vi "Init from Ref.vi"(8 "error in":errorcluster, 10 "Cell Ref":refnum<k24>, 11 "Image in":refnum<class "Image.lvclass">) -> (0 "error out":errorcluster, 3 "Image out":refnum<class "Image.lvclass">)   [LabVIEW 2023, in "SourceGrid.lvlib" / "Image.lvclass"]
uses:
  Image.lvclass
  D:/git/Sourcegrid-LabVIEW/dll/SourceGrid.dll
  dll/SourceGrid.dll
  Cell/Cell.lvclass
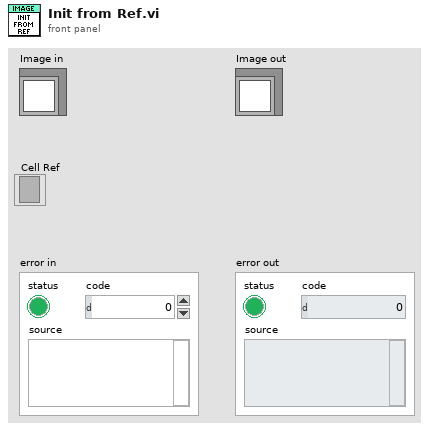
[diagram p1: front panel]
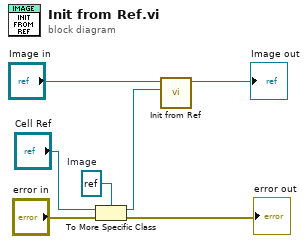
[diagram p0: block diagram]
diagram:
  w1 = refnum<k24> refnum  # Image
  n1 = To More Specific Class(target class=w1, reference="Cell Ref", error in="error in") -> (specific class reference=w2:refnum<k24>, error out=→"error out":errorcluster)
  n2 = call-parent "Init from Ref.vi"("Cell"=w2, "Cell in"="Image in") -> ("Cell out"=→"Image out":refnum<class "Image.lvclass">)  [unwired: 8 in, 1 out]
